vi "initialize.vi"(8 "error in (no error)":errorcluster, 9 "Commands":T1[](array[typedef]), 10 "Properties":T2[](array[typedef]), 11 "name":string) -> (0 "error out":errorcluster, 3 "Relay out":refnum<class "Relay.lvclass">)   [LabVIEW 2015, in "SLSC Switch.lvlib" / "Relay.lvclass"]
uses:
  Relay.lvclass
  Property.ctl
  Command.ctl
  Relay.lvclass/Relay.ctl
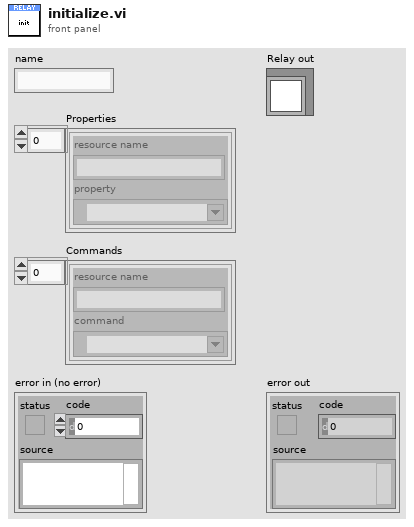
[diagram p1: front panel]
types:
  T1 = typedef "SLSC Switch.lvlib/Relay.lvclass/Command.ctl" = cluster{"resource name":string, "command":refnum<k21>}
  T2 = typedef "SLSC Switch.lvlib/Relay.lvclass/Property.ctl" = cluster{"resource name":string, "property":refnum<k21>}
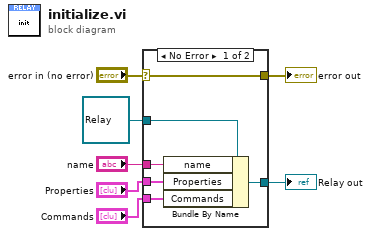
[diagram p0: block diagram]
diagram:
  n1 = case shown="No Error" "error in (no error)" {
    selector: "error in (no error)" -> [w8 w15]
    tunnel: [w8 w15] -> w6
    tunnel: [w9 w14] -> w4
    tunnel: refnum<class "Relay.lvclass"> refnum ("Relay in") -> [w13 w14]
    tunnel: "name" -> [w12 _]
    tunnel: "Properties" -> [w11 _]
    tunnel: "Commands" -> [w10 _]
    frame No Error {
      n2 = Bundle By Name(cluster=w13, "name"=w12, "Properties"=w11, "Commands"=w10) -> (w9:refnum<class "Relay.lvclass">)
    }
    frame Error {
    }
  }
  "error out" <- w6
  "Relay out" <- w4
